vi "Compare Calls.vi"(8 "error in (no error)":errorcluster, 9 "VI Call 2":refnum<class "VI Call.lvclass">, 10 "VI Call 1":refnum<class "VI Call.lvclass">, 11 "Ignore Inputs Comparator in":refnum<class "Any Inputs Comparator.lvclass">) -> (0 "error out":errorcluster, 1 "Description":string, 2 "Equal?":bool)   [LabVIEW 2020, in "Any Inputs Comparator.lvclass"]
uses:
  Any Inputs Comparator.lvclass
  Core/VI Call/VI Call.lvclass
  <vilib>/AdvancedString/1D String Array to Delimited String.vi
  Core/Comparator/Describe Variant.vi
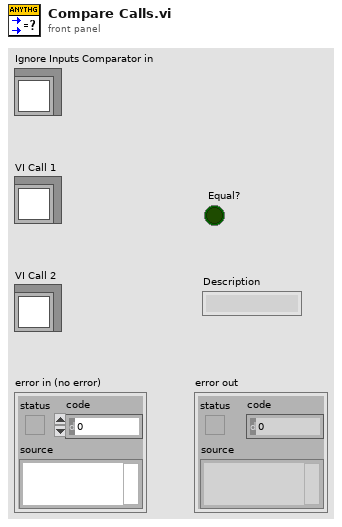
[diagram p1: front panel]
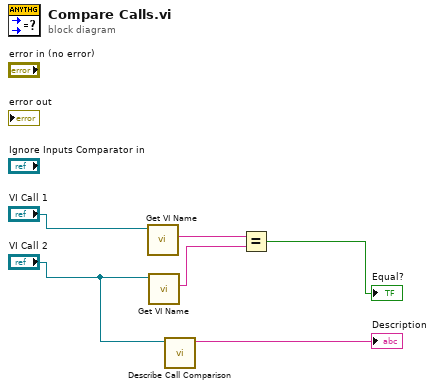
[diagram p0: block diagram]
diagram:
  n1 = call-dynamic "Get VI Name.vi"("VI Call In"="VI Call 1") -> ("VI Name"=w6:string)  [unwired: 10 in]
  n2 = call-dynamic "Get VI Name.vi"("VI Call In"="VI Call 2") -> ("VI Name"=w5:string)  [unwired: 10 in]
  n3 = call "Describe Call Comparison.vi"("VI Call in"="VI Call 2") -> ("delimited string"=→"Description":string)  [unwired: 10 in]
  n4 = Equal?(x=w6, y=w5) -> (x = y?=→"Equal?":bool)
